vi "Test Find Class from Path.vi"(8 "error in (no error)":errorcluster, 11 "Test Finder Test in":refnum<class "Finder Test.lvclass">) -> (0 "error out":errorcluster, 3 "Test Finder Test out":refnum<class "Finder Test.lvclass">)   [LabVIEW 2020, in "LUnit Tests.lvlib" / "Finder Test.lvclass"]
uses:
  Finder Test.lvclass
  Finder Test.lvclass/Finder Test.ctl
  source/Framework/Helper Classes/Test Finder/Test Finder.lvclass
  Test Dummys/Test Test Case/Test Test Case.lvclass
  <vilib>/Astemes/LUnit/Test Case.lvclass
  C:/Program Files (x86)/National Instruments/LabVIEW 2020/vi.lib/Astemes/LUnit/Test Case.lvclass
  C:/Git/astemes-lunit/tests/Test Finder/Finder Test.lvclass
  C:/Git/astemes-lunit/source/Framework/Test Case/LUnit Test Case.lvclass
  C:/Git/astemes-lunit/tests/Test Dummys/Test Test Case/Test Test Case.lvclass
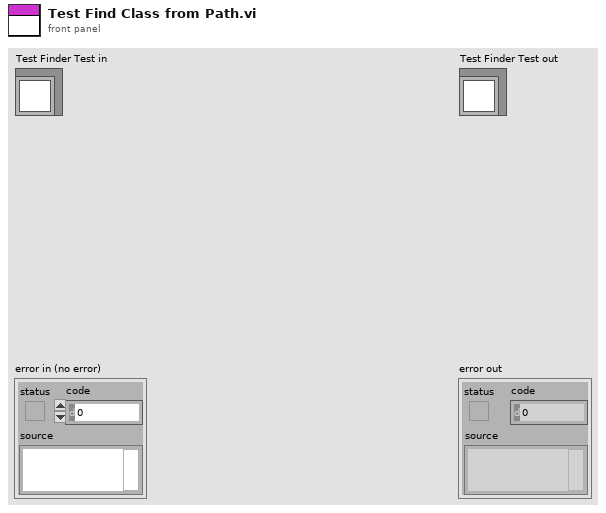
[diagram p1: front panel]
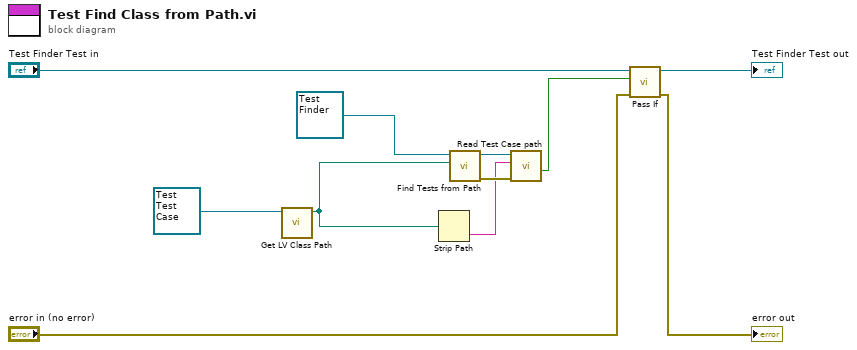
[diagram p0: block diagram]
diagram:
  n1 = call <vilib>:"Get LV Class Path.vi"("object"=refnum<class "Test Test Case.lvclass"> refnum ("Test Test Case.lvclass")) -> ("class path"=w3:path)  [unwired: 9 in, 1 out]
  n2 = Strip Path(path=w3) -> (name=w2:string)  [unwired: 1 out]
  n3 = call-dynamic "Find Tests from Path.vi"("Project or Class Path"=w3, "Test Case Finder In"=refnum<class "Test Finder.lvclass"> refnum) -> ("error out"=w6:errorcluster, "Test Case Finder Out"=w7:refnum<class "Test Finder.lvclass">)  [unwired: 8 in]
  n4 = call "Read Test Case path.vi"("error in (no error)"=w6, "Test Case Name"=w2, "Test Case Finder In"=w7) -> ("found?"=w1:bool)  [unwired: 5 in, 3 out]
  n5 = call <vilib>:"Pass If.vi"("error in (no error)"="error in (no error)", "Pass?"=w1, "LUnit Test Case In"="Test Finder Test in") -> ("error out"=→"error out":errorcluster, "LUnit Test Case Out"=→"Test Finder Test out":refnum<class "Finder Test.lvclass">)  [unwired: 7 in]
